vi "New1000.vi"   [LabVIEW 2013]
uses:
  <vilib>/Heliosphere Research LLC/Advanced Plotting Toolkit/api_core/NewPlotProperties.ctl
  <vilib>/Heliosphere Research LLC/Advanced Plotting Toolkit/typedefs/PlotColor.ctl
  <vilib>/Heliosphere Research LLC/Advanced Plotting Toolkit/api_core/NewPlotType.ctl
  <vilib>/Heliosphere Research LLC/Advanced Plotting Toolkit/Advanced Plotting Toolkit.lvlib
types:
  T1 = typedef "Advanced Plotting Toolkit.lvlib/NewPlotType.ctl" = enum16{"Rectangular Axes", "Polar Axes"}
  T2 = typedef "Advanced Plotting Toolkit.lvlib/NewPlotProperties.ctl" = cluster{"Background Color":T3, "Axis Background":T3, "Left Margin":dbl, "Right Margin":dbl, "Bottom Margin":dbl, "Top Margin":dbl, "Aspect Ratio":dbl}
  T3 = typedef "Advanced Plotting Toolkit.lvlib/PlotColor.ctl" = u32
  T4 = typedef "Advanced Plotting Toolkit.lvlib/PlotID.ctl" = i32
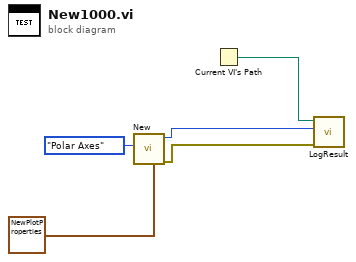
[diagram p0: block diagram]
diagram:
  n1 = call <vilib>:"New.vi"("Properties"=T2 {"Background Color"=2147483647, "Axis Background"=2147483647, "Left Margin"=nan, "Right Margin"=nan, "Bottom Margin"=nan, "Top Margin"=nan, "Aspect Ratio"=nan} ("New Plot Properties"), "Plot Type"=NewPlotType."Polar Axes") -> ("error out"=w3:errorcluster, "Plot ID"=w4:T4)  [unwired: 8 in]
  n2 = Current VI's Path() -> (path=w5:path)
  n3 = call "LogResult.vi"("Test Result"=w3, "Test Artifact"=w4, "VI Path"=w5) -> ()  [unwired: 9 in]
